vi "set Port Name.vi"(10 "port_name":string, 11 "port_num":i32) -> ()   [LabVIEW 2016, in "dxl_x86_c.lvlib"]
doc: "WINDECLSPEC void setPortName (int port_num, const char* port_name);"
uses:
  dxl_x86_c.lvlib
  dxl_x86_c.dll
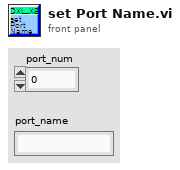
[diagram p1: front panel]
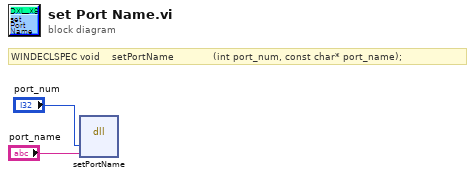
[diagram p0: block diagram]
diagram:
  # "WINDECLSPEC void    setPortName             (int port_num, const char* port_name);"
  n1 = dll-call lib="C:/Users/Platform/Desktop/DynamixelSDK/labview/dxl_x86_c.lvlib/dxl_x86_c.*" fn="setPortName"("port_num"="port_num", "port_name"="port_name") -> ()  [unwired: 6 in, 2 out]
